vi "Core Logic.vi"(0 "Measurement Context In":refnum<class "Measure Call Context.lvclass">, 5 "Measurement Configuration":T2={"Quick Power Down"=FALSE, "Pin Name"=[], "Source Mode"=[], "Start Value"=[], "Target Value"=[], "Compliance Limit"=[], "Sense Mode"=[], "Default Ramp Rate"=[], "Ramp Rate"=[], "Start Delay"=[], "Relative To"=[], "Transient Response"=[], "Data Capture"=FALSE, "Power line frequency"=1} {"Power line frequency" items=["50 Hz", "60 Hz"]; "Start Value" format="%#_6p"; "Transient Response" items=["Slow", "Normal", "Fast"]; "Sense Mode" items=["Local Sense", "Remote Sense"]; "Relative To" items=["Power sequence start", "Previous source start", "Previous source end"]; "Target Value" format="%#_6p"; "Source Mode" items=["DC Voltage", "DC Current"]; "Start Delay" format="%#_6p"; "Compliance Limit" format="%#_6p"; "Ramp Rate" format="%#_6p"}, 11 "error in":errorcluster) -> (4 "Measurement Context Out":refnum<class "Measure Call Context.lvclass">, 6 "Measurement Results":T1, 15 "error out":errorcluster)   [LabVIEW 2024, in "devicePowerSequencerCoreLogic.lvlib"]
doc: "Use this template to build a producer/consumer design pattern. Use this template when you need to execute a process, such as data analysis, when a data source, such as a triggered acquisition, produces data at an uneven rate and you need to execute the process when the data becomes available."
uses:
  devicePowerSequencerCoreLogic.lvlib
  Measurement Configuration.ctl
  controls/Source Mode.ctl
  controls/Sense Mode.ctl
  controls/Relative To.ctl
  controls/Transient Response.ctl
  controls/Power line frequency.ctl
  Measurement Results.ctl
  <vilib>/Plug-In SDKs/Measurements/Measure Call Context/Measure Call Context.lvclass
  controls/Data Cluster.ctl
  <vilib>/Plug-In SDKs/Clients/Session Management V1/Session Reservation/Session Reservation.lvclass
  controls/Channel Name.ctl
  controls/Software Flags.ctl
  controls/Ramp Configurations.ctl
  controls/Error Info.ctl
  controls/Measurements.ctl
  controls/Voltage and Current Measurements.ctl
  controls/Log Configurations.ctl
  <instrlib>/niDCPower/nidcpower.llb/niDCPower Wait For Event - Event.ctl
  subVIs/Form Error Message.vi/4da3fa3f-d6a2-4c6b-9c9c-fc44bca91f7b.vi
  <vilib>/Plug-In SDKs/Measurements/Measure Call Context/Reserve Sessions - NPin.vi
  <vilib>/Plug-In SDKs/Sessions/niDCPower/Initialize Sessions - NSess.vi
  <vilib>/Plug-In SDKs/Measurements/Measure Call Context/Accessor/Is Canceled.vi
  Device Power Sequencer.lvlib
  <vilib>/Plug-In SDKs/Sessions/niDCPower/NI Session Management niDCPower.lvlib
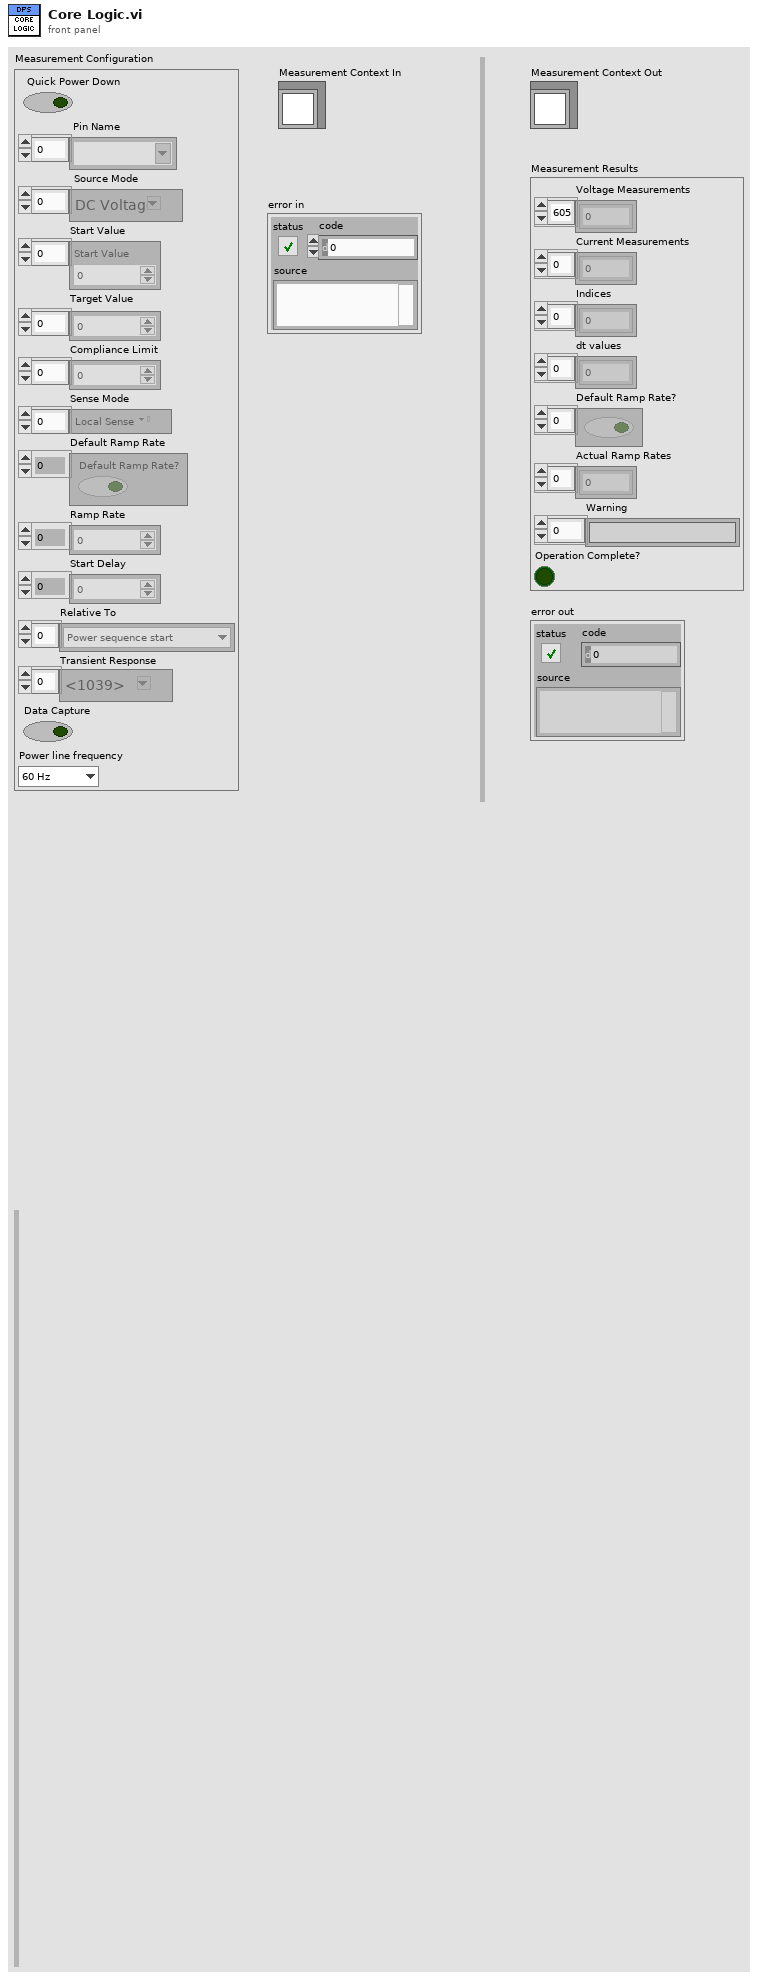
[diagram p1: front panel]
types:
  T1 = typedef "Device Power Sequencer.lvlib/Measurement Results.ctl" = cluster{"Voltage Measurements":dbl[], "Current Measurements":dbl[], "Indices":i32[], "dt values":dbl[], "Default Ramp Rate?":bool[], "Actual Ramp Rates":dbl[], "Warning":string[], "Operation Complete?":bool}
  T2 = typedef "Device Power Sequencer.lvlib/Measurement Configuration.ctl" = cluster{"Quick Power Down":bool, "Pin Name":string[], "Source Mode":T3[], "Start Value":dbl[], "Target Value":dbl[], "Compliance Limit":dbl[], "Sense Mode":T4[], "Default Ramp Rate":bool[], "Ramp Rate":dbl[], "Start Delay":dbl[], "Relative To":T5[], "Transient Response":T6[], "Data Capture":bool, "Power line frequency":T7}
  T3 = typedef "Device Power Sequencer.lvlib/Source Mode.ctl" = i32
  T4 = typedef "Device Power Sequencer.lvlib/Sense Mode.ctl" = i32
  T5 = typedef "Device Power Sequencer.lvlib/Relative To.ctl" = u32
  T6 = typedef "Device Power Sequencer.lvlib/Transient Response.ctl" = i32
  T7 = typedef "Device Power Sequencer.lvlib/Power line frequency.ctl" = u32
  T8 = typedef "devicePowerSequencerCoreLogic.lvlib/Data Cluster.ctl" = cluster{"session reservation":refnum<class "Session Reservation.lvclass">, "measurement context":refnum<class "Measure Call Context.lvclass">, "Measurement Configuration":T2, "Measurement Results":T1, "Channel Settings":T9, "Software Flags":T10, "Ramp Configurations":T11, "Error Info":T12, "Measurements":T13, "Log":T15}
  T9 = typedef "devicePowerSequencerCoreLogic.lvlib/Channel Name.ctl" = cluster{"Channel Name":string[], "Channel Number":string[], "Instrument handle":refnum<k15>[], "Session Exists?":bool[], "Session.name":string[]}
  T10 = typedef "devicePowerSequencerCoreLogic.lvlib/Software Flags.ctl" = cluster{"Initialize Complete?":bool, "Configuration Complete?":bool, "Run Complete?":bool, "Output Complete?":bool, "Safe Power Down In Progress?":bool, "Power Up Operation?":bool, "Canceled?":bool, "Session exists?":bool[], "Advanced Seq Created?":bool[], "Initiated?":bool[], "Unsupported Ramp?":bool[], "Compliance Reached?":bool[], "PowerUp?":bool, "Unsupported Start Delay?":bool[]}
  T11 = typedef "devicePowerSequencerCoreLogic.lvlib/Ramp Configurations.ctl" = cluster{"Minimum Sequence dt(s)":dbl[], "Sequence Delta(s)":dbl[], "Number of steps":i32[], "Actual Ramp Rate(Unit/S)":dbl[], "Total Sequence Time":dbl, "Rising Period":dbl[], "Accumulative Start Delay(s)":dbl[], "Temporary Target Level":dbl[], "Start Level":dbl[], "Measure Period":dbl, "Compliance Skip Duration":dbl[], "Max Sequence Period Index":i32, "Compliance Check Duration":dbl}
  T12 = typedef "devicePowerSequencerCoreLogic.lvlib/Error Info.ctl" = cluster{"Error Occurred?":bool, "Warning List":string[], "Error Phase":string, "Error Code":i32, "error":errorcluster, "Error List":string[], "Custom Error?":bool}
  T13 = typedef "devicePowerSequencerCoreLogic.lvlib/Measurements.ctl" = cluster{"Measurements":T14[], "Calculated Ramp Rate":dbl[], "Default RampRate?":bool[], "Aperture Time":dbl[]}
  T14 = typedef "devicePowerSequencerCoreLogic.lvlib/Voltage and Current Measurements.ctl" = cluster{"Voltage Measurements":dbl[], "Current Measurements":dbl[], "Compliance":bool[]}
  T15 = typedef "devicePowerSequencerCoreLogic.lvlib/Log Configurations.ctl" = cluster{"User Event":refnum<user-event>, "Measure Complete":bool, "Log File Ref.":refnum<file>, "Log Data?":bool, "Async Log Ref.":refnum<vi>}
  T16 = cluster{"Measurment":cluster{"Voltage":dbl[], "Current":dbl[]}[], "Measure Complete?":bool}
  T17 = typedef "niDCPower Wait For Event - Event.ctl" = i32
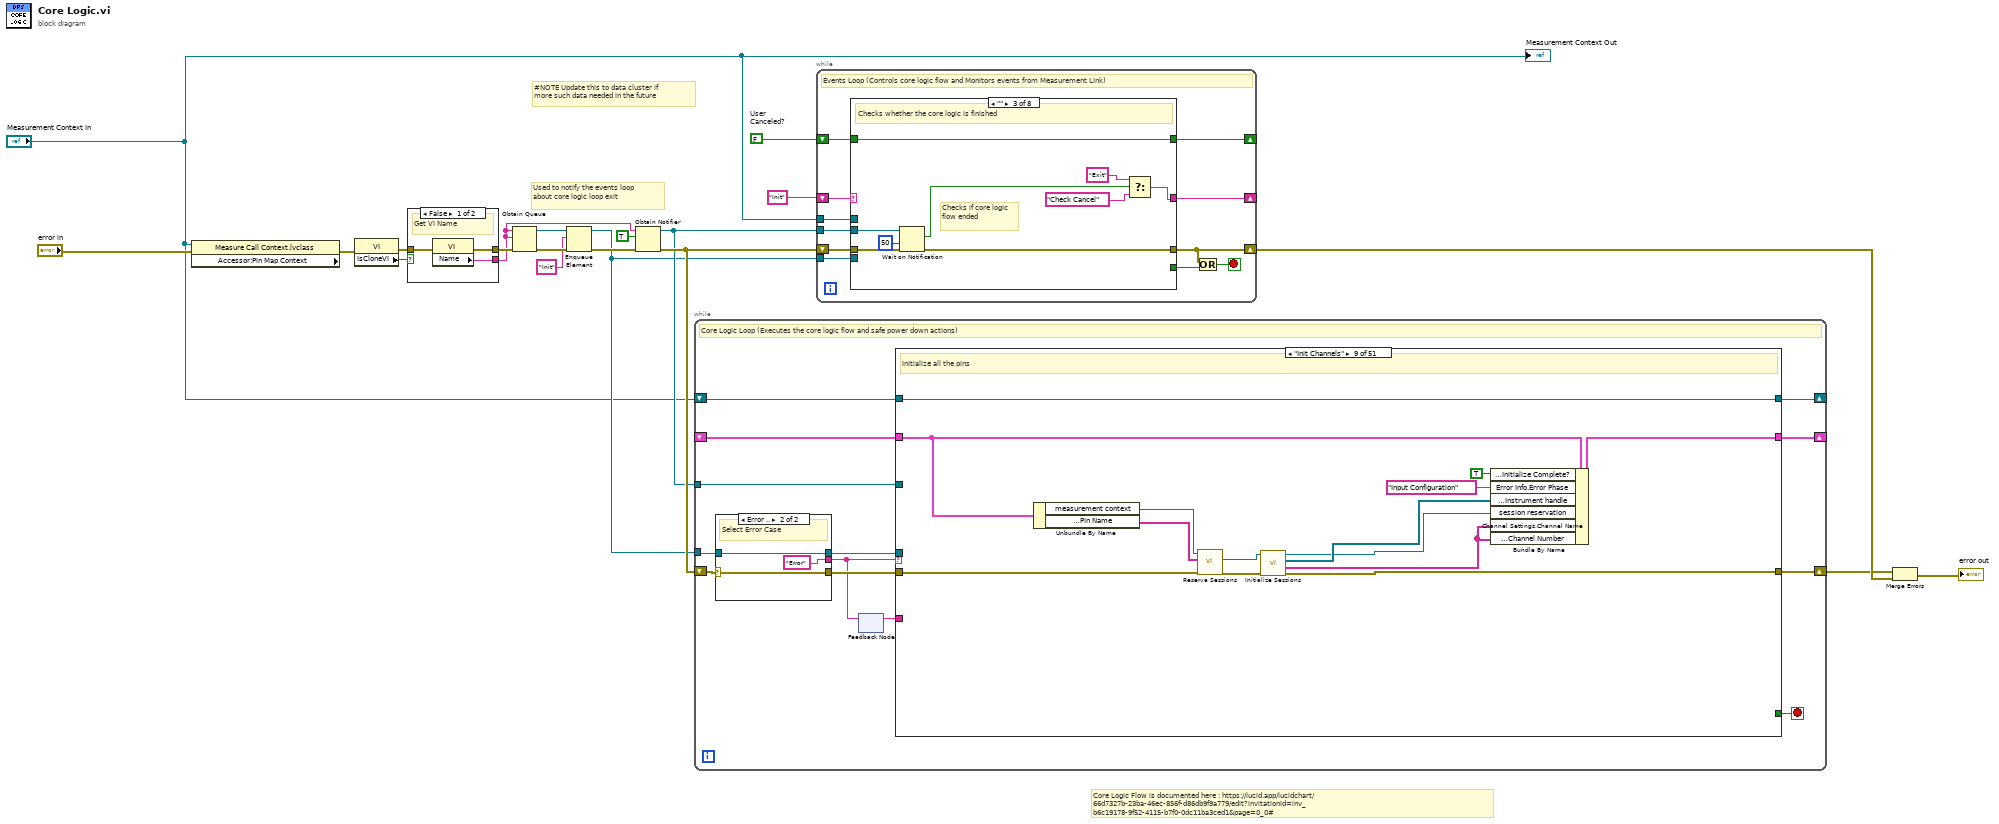
[diagram p0: block diagram]
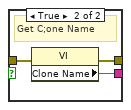
[diagram p2: hidden frame]
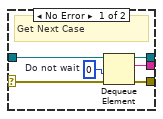
[diagram p3: hidden frame]
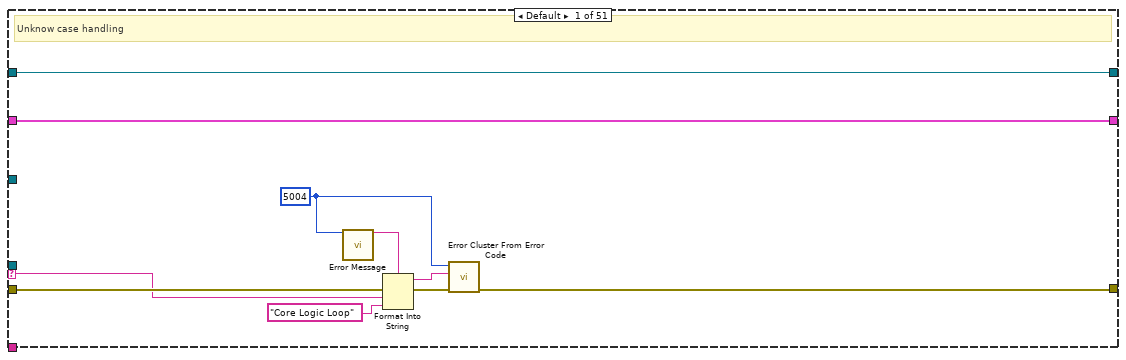
[diagram p4: hidden frame]
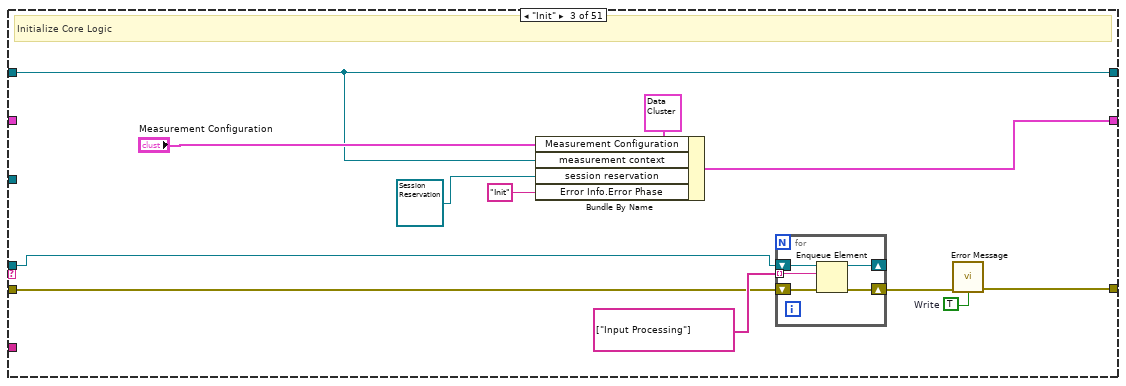
[diagram p6: hidden frame]
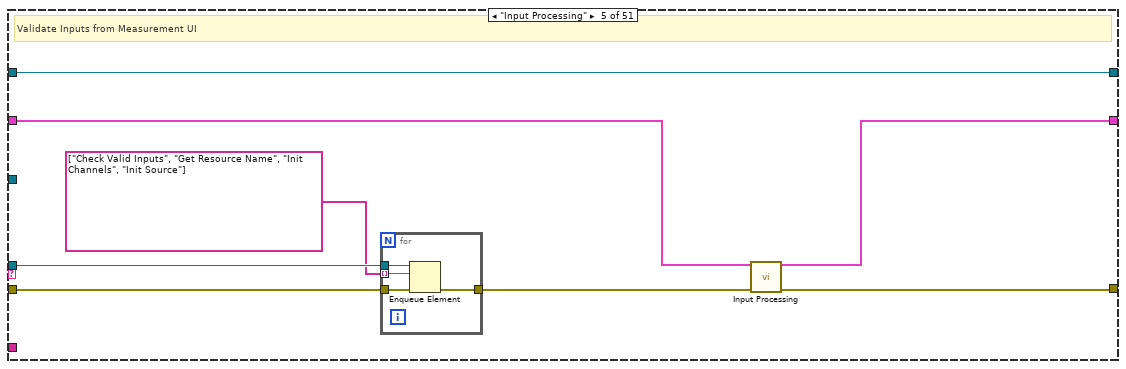
[diagram p8: hidden frame]
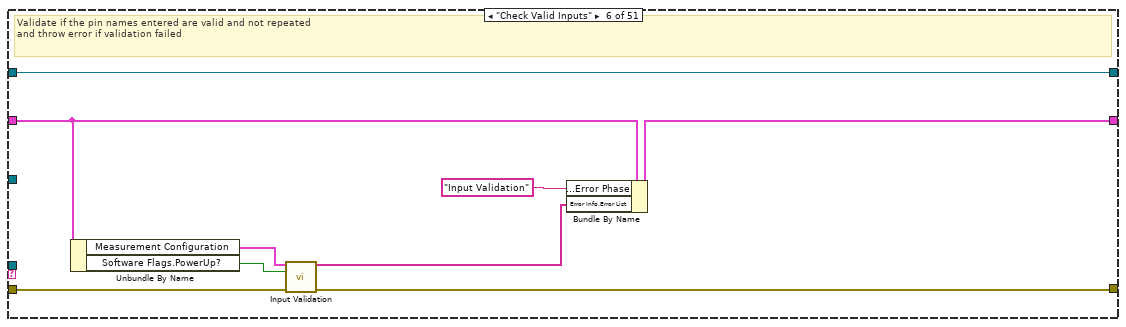
[diagram p9: hidden frame]
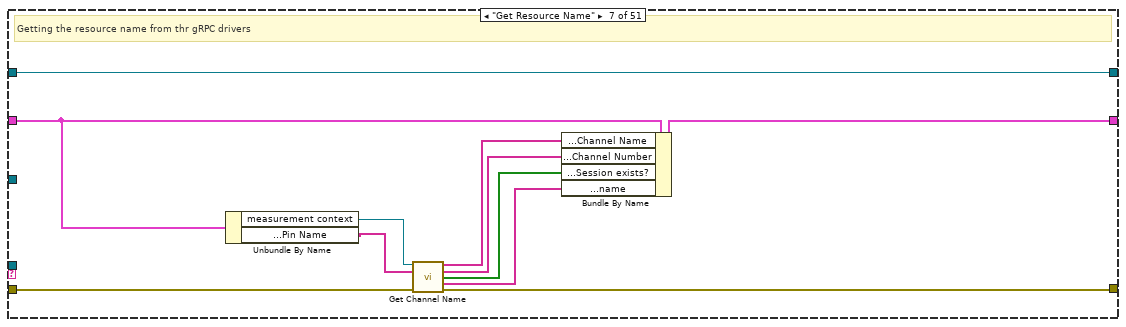
[diagram p10: hidden frame]
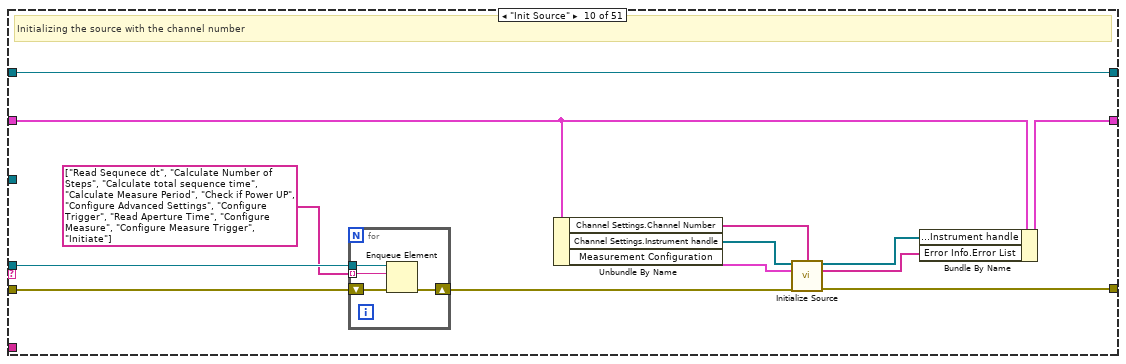
[diagram p12: hidden frame]
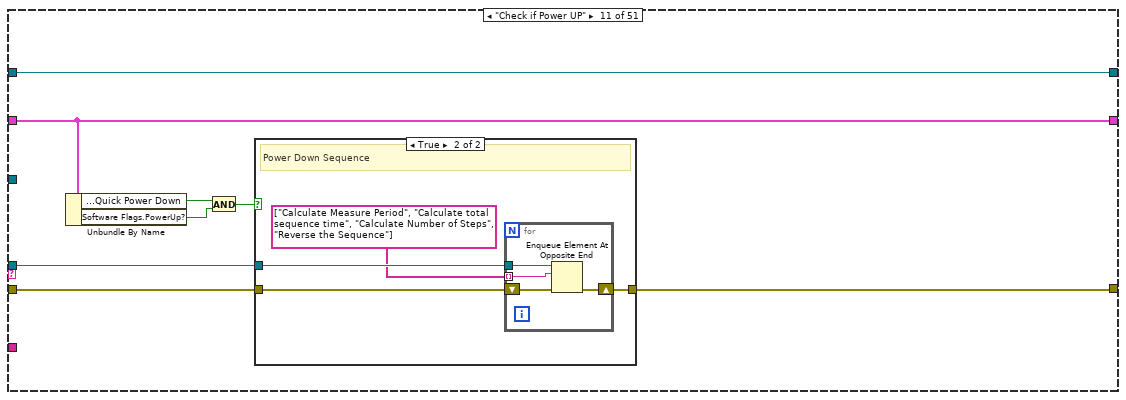
[diagram p13: hidden frame]
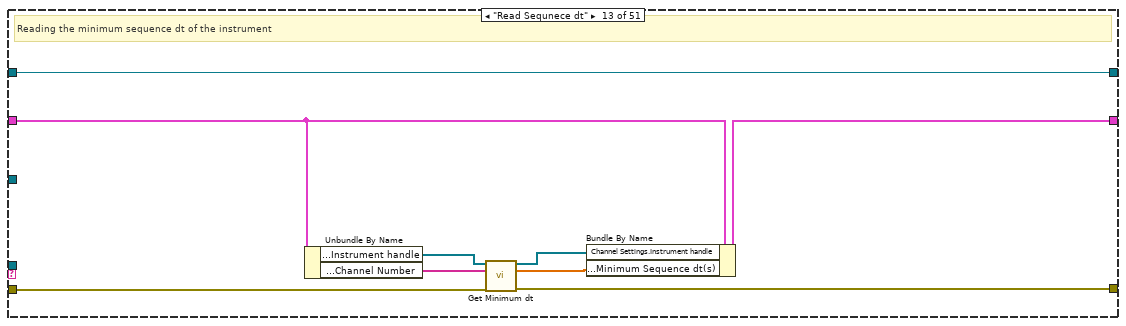
[diagram p16: hidden frame]
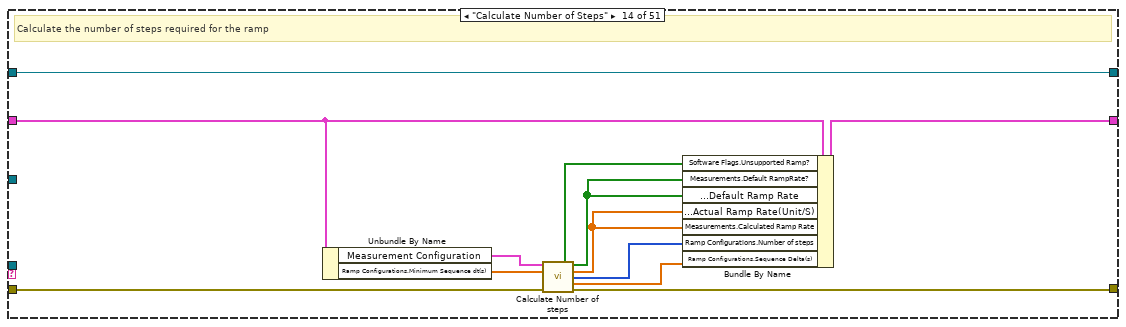
[diagram p17: hidden frame]
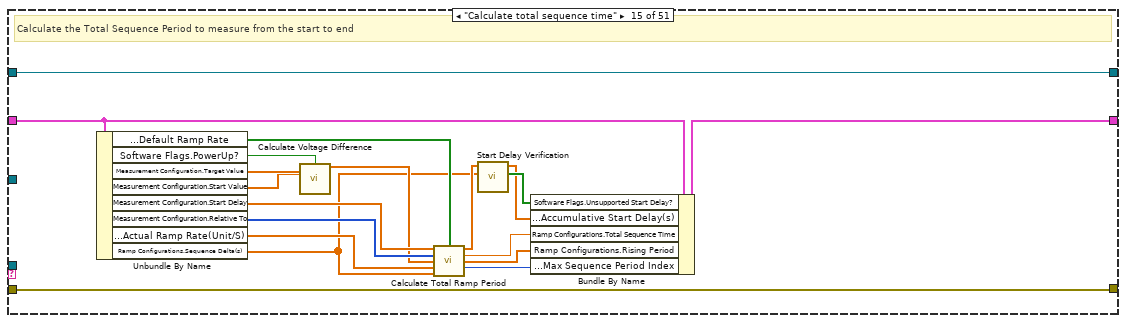
[diagram p18: hidden frame]
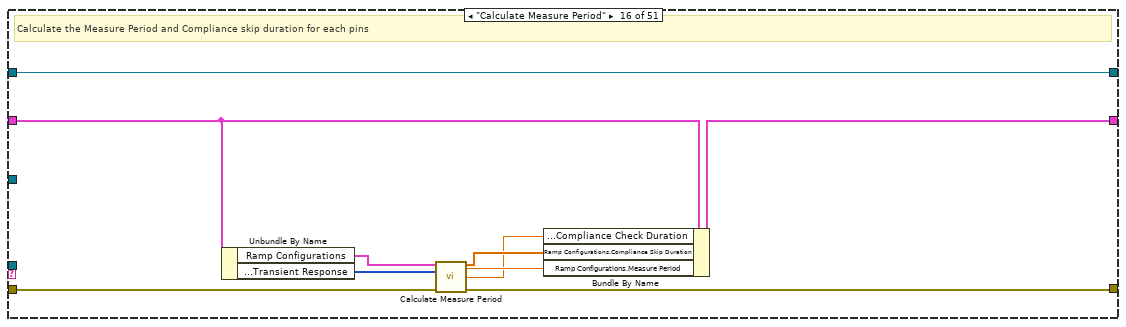
[diagram p19: hidden frame]
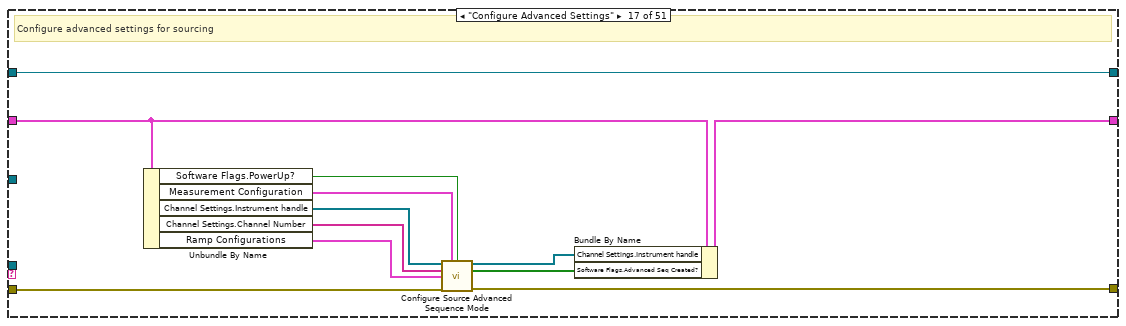
[diagram p20: hidden frame]
diagram:
  w10 = FALSE  # User Canceled?
  # "#NOTE Update this to data cluster if more such data needed in the future"
  # "Core Logic Flow is documented here : https://lucid.app/lucidchart/66d7327b-23ba-46ec-856f-d86db9f9a779/edit?invitationId=inv_b6c19178-9f52-4115-b7f0-0dc11ba3ced1&page=0_0#"
  # "Used to notify the events loop about core logic loop exit"
  n1 = property class="Measure Call Context.lvclass" props=["Accessor:Pin Map Context"](reference="Measurement Context In", error in="error in") -> (error out=w2:errorcluster)  [unwired: 2 out]
  n2 = property class="VI"(error in=w2) -> (error out=w6:errorcluster, "IsCloneVI"=w5:bool)  [unwired: 1 in, 1 out]
  n3 = case shown="False" w5 {
    tunnel: [w23 w25] -> w20
    tunnel: [w22 w24] -> w7
    tunnel: w6 -> [w21 w26]
    frame False {
      # "Get VI Name"
      n4 = property class="VI"(error in=w21) -> (error out=w23:errorcluster, "Name"=w22:string)  [unwired: 1 in, 1 out]
    }
    frame True {
      # "Get C;one Name"
      n5 = property class="VI"(error in=w26) -> (error out=w25:errorcluster, "Clone Name"=w24:string)  [unwired: 1 in, 1 out]
    }
  }
  n6 = Obtain Queue(name (unnamed)=w7, element data type=w7, error in (no error)=w20) -> (queue out=w9:refnum<queue>, error out=w19:errorcluster)  [unwired: 2 in, 1 out]
  n7 = Enqueue Element(queue=w9, element="Init" ("State In"), error in (no error)=w19) -> (queue out=w8:refnum<queue>, error out=w14:errorcluster)  [unwired: 1 in, 1 out]
  n8 = Obtain Notifier(name (unnamed)=w7, notification data type=TRUE, error in (no error)=w14) -> (notifier out=w12:refnum<notifier>, error out=w13:errorcluster)  [unwired: 1 in, 1 out]
  n9 = while {
    shift-right: [w36] -> w4
    shift-left: w13 -> [w38]
    shift-right: [w35] -> _
    shift-left: _ -> [w34]
    tunnel: w12 -> [w33]
    tunnel: w8 -> [w32]
    shift-right: [w27] -> _
    shift-left: "Measurement Context In" -> [w28]
    stop <- w39 stop-if-true
    # "Core Logic Loop (Executes the core logic flow and safe power down actions)"
    n10 = case shown="Error .." w38 {
      selector: w38 -> [w45 w48]
      tunnel: [w44 w48] -> w37
      tunnel: [w43 "Error"] -> w30
      tunnel: w32 -> [w42 w47]
      tunnel: [w40 w47] -> w31
      frame No Error {
        w41 = 0  # Do not wait
        # "Get Next Case"
        n11 = Dequeue Element(queue=w42, timeout in ms (-1)=w41, error in (no error)=w45) -> (queue out=w40:refnum<queue>, element=w43:string, error out=w44:errorcluster)  [unwired: 1 out]
      }
      frame Error {
        # "Select Error Case"
      }
    }
    n12 = feedback-in #1(w30) -> ()
    n13 = feedback #1() -> (w29:string)  [unwired: 1 in]
    n14 = case shown="\"Init Channels\"" w30 {
      selector: w30 -> [w54 _ _ _ _ _ _ _ _ _ _ _ _ _ _ _ _ _ _ _ _ _ _ _ _ _ _ _ _ _ _ _ _ _ _ _ _ _ _ _ _ _ _ _ _ _ _ _ _ _ _]
      tunnel: [_ _ _ _ _ _ _ _ _ _ _ _ _ _ _ _ _ _ _ _ _ _ _ _ _ _ _ _ _ _ _ _ _ _ _ _ _ _ _ _ _ _ _ _ _ _ _ _ _ _ w738] -> w39
      tunnel: w37 -> [w58 w61 w63 w81 w89 w99 w111 w116 w128 w140 w154 w167 w173 w183 w207 w211 w223 w231 w239 w244 w255 w264 w271 w275 w281 w285 w300 w310 w323 w335 w354 w370 w387 w405 w420 w426 w437 w453 w462 w482 w491 w508 w514 w527 w561 w571 w591 w610 w616 w706 w730]
      tunnel: [w56 w61 w67 w81 w84 w100 w112 w116 w129 w137 w152 w167 w174 w182 w207 w210 w224 w232 w239 w243 w256 w265 w271 w274 w280 w284 w297 w310 w318 w335 w360 w370 w383 w411 w420 w422 w438 w453 w461 w483 w486 w509 w514 w520 w561 w572 w592 w610 w622 w705 w717] -> w36
      tunnel: [w57 w60 w71 w80 w85 w98 w110 w115 w127 w142 w155 w166 w172 w186 w203 w214 w222 w236 w238 w245 w258 w268 w270 w273 w279 w287 w291 w309 w327 w334 w342 w367 w382 w413 w419 w425 w436 w452 w464 w480 w493 w511 w513 w532 w560 w570 w595 w609 w617 w704 w719] -> w35
      tunnel: w34 -> [w57 w60 _ w80 w86 w102 w113 w115 w130 w143 w155 w166 w176 w181 w206 w217 w229 w236 w238 w246 w262 w268 w270 w276 w282 w288 w298 w309 w313 w334 w343 w369 w384 w409 w419 w431 w441 w452 w459 w481 w498 w511 w513 w533 w560 w568 w601 w609 w624 w708 w719]
      tunnel: w33 -> [_ _ _ _ _ _ _ _ _ _ _ _ _ _ _ _ _ _ _ _ _ _ _ _ _ _ _ _ _ _ _ _ _ _ _ _ _ _ _ _ _ _ _ _ _ _ _ _ _ _ w736]
      tunnel: w31 -> [_ _ w72 _ w88 _ _ _ _ w141 w153 _ _ _ _ _ _ _ _ _ _ _ _ _ _ w286 _ _ w325 _ w359 _ _ w407 _ _ _ _ w460 _ _ _ _ w529 _ w574 _ _ w621 _ w733]
      tunnel: w29 -> [_ _ _ _ _ _ _ _ _ _ _ _ _ _ _ _ _ _ _ _ _ _ _ _ _ _ _ _ _ _ _ _ _ _ _ _ _ _ _ _ _ _ _ _ _ _ _ _ w612 _ _]
      tunnel: w28 -> [w49 w59 w64 w79 w82 w94 w105 w114 w123 w132 w148 w165 w168 w177 w189 w208 w218 w230 w237 w240 w251 w263 w269 w272 w277 w283 w289 w308 w311 w333 w336 w365 w374 w401 w418 w421 w433 w451 w454 w479 w484 w499 w512 w515 w559 w562 w581 w608 w611 w700 w715]
      tunnel: [w49 w59 w64 w79 w82 w94 w105 w114 w123 w132 w148 w165 w168 w177 w189 w208 w218 w230 w237 w240 w251 w263 w269 w272 w277 w283 w289 w308 w311 w333 w336 w365 w374 w401 w418 w421 w433 w451 w454 w479 w484 w499 w512 w515 w559 w562 w581 w608 w611 w700 w715] -> w27
      frame Default {
        w51 = 5004 ("error code (0)")
        # "Unknow case handling"
        n15 = call "Error Message.vi"("Error Code"=w51) -> ("Error Message"=w50:string)  [unwired: 12 in, 2 out]
        n16 = Format Into String(format string=w50, error in=w58, w54, "Core Logic Loop" ("input 2")) -> (resulting string=w53:string, error out=w55:errorcluster)  [unwired: 1 in]
        n17 = call <vilib>:"Error Cluster From Error Code.vi"("error in (no error)"=w55, "error message (\"\")"=w53, "error code (0)"=w51) -> ("error out"=w56:errorcluster)  [unwired: 6 in]
      }
      frame "----------------- INITIALIZE -----------------" {
      }
      frame "Init" {
        w70 = TRUE  # Write
        # "Initialize Core Logic"
        n18 = Bundle By Name(cluster=T8 {"session reservation"=refnum, "measurement context"=refnum, "Measurement Configuration"={"Quick Power Down"=FALSE, "Pin Name"=[], "Source Mode"=[], "Start Value"=[], "Target Value"=[], "Compliance Limit"=[], "Sense Mode"=[], "Default Ramp Rate"=[], "Ramp Rate"=[], "Start Delay"=[], "Relative To"=[], "Transient Response"=[], "Data Capture"=FALSE, "Power line frequency"=1}, "Measurement Results"={"Voltage Measurements"=[], "Current Measurements"=[], "Indices"=[], "dt values"=[], "Default Ramp Rate?"=[], "Actual Ramp Rates"=[], "Warning"=[], "Operation Complete?"=FALSE}, "Channel Settings"={"Channel Name"=[], "Channel Number"=[], "Instrument handle"=[], "Session Exists?"=[], "Session.name"=[]}, "Software Flags"={"Initialize Complete?"=FALSE, "Configuration Complete?"=FALSE, "Run Complete?"=FALSE, "Output Complete?"=FALSE, "Safe Power Down In Progress?"=FALSE, "Power Up Operation?"=FALSE, "Canceled?"=FALSE, "Session exists?"=[], "Advanced Seq Created?"=[], "Initiated?"=[], "Unsupported Ramp?"=[], "Compliance Reached?"=[], "PowerUp?"=FALSE, "Unsupported Start Delay?"=[]}, "Ramp Configurations"={"Minimum Sequence dt(s)"=[], "Sequence Delta(s)"=[], "Number of steps"=[], "Actual Ramp Rate(Unit/S)"=[], "Total Sequence Time"=0.0, "Rising Period"=[], "Accumulative Start Delay(s)"=[], "Temporary Target Level"=[], "Start Level"=[], "Measure Period"=0.0, "Compliance Skip Duration"=[], "Max Sequence Period Index"=0, "Compliance Check Duration"=0.0}, "Error Info"={"Error Occurred?"=FALSE, "Warning List"=[], "Error Phase"="", "Error Code"=5100, "error"={"status"=FALSE, "code"=0, "source"=""}, "Error List"=[], "Custom Error?"=FALSE}, "Measurements"={"Measurements"=[], "Calculated Ramp Rate"=[], "Default RampRate?"=[], "Aperture Time"=[]}, "Log"={"User Event"=refnum, "Measure Complete"=FALSE, "Log File Ref."=refnum, "Log Data?"=FALSE, "Async Log Ref."=refnum}} ("Data Cluster"), "Measurement Configuration"="Measurement Configuration", "measurement context"=w64, "session reservation"=refnum<class "Session Reservation.lvclass"> refnum, "Error Info.Error Phase"="Init") -> (w71:T8)
        n19 = for {
          shift-right: [w76] -> w69
          shift-left: w63 -> [w78]
          shift-right: [w75] -> _
          shift-left: w72 -> [w77]
          tunnel: string[] ["Input Processing"] -> [w74] mode=indexing
          n20 = Enqueue Element(queue=w77, element=w74, error in (no error)=w78) -> (queue out=w75:refnum<queue>, error out=w76:errorcluster)  [unwired: 1 in, 1 out]
        }
        n21 = call "Error Message.vi"("error in (no error)"=w69, "ReadError?F:T"=w70) -> ("error out"=w67:errorcluster)  [unwired: 11 in, 2 out]
      }
      frame "---------------------VALIDATION---------------------" {
      }
      frame "Input Processing" {
        # "Validate Inputs from Measurement UI"
        n22 = for {
          tunnel: string[] ["Check Valid Inputs", "Get Resource Name", "Init Channels", "Init Source"] ("State In") -> [w92] mode=indexing
          tunnel: w88 -> [w90]
          tunnel: w89 -> [w91]
          tunnel: [w93] -> w83
          n23 = Enqueue Element(queue=w90, element=w92, error in (no error)=w91) -> (error out=w93:errorcluster)  [unwired: 1 in, 2 out]
        }
        n24 = call "Input Processing.vi"("Data Cluster"=w86, "error in (no error)"=w83) -> ("Data Cluster OUT"=w85:T8, "error out"=w84:errorcluster)  [unwired: 12 in]
      }
      frame "Check Valid Inputs" {
        # "Validate if the pin names entered are valid and not repeated\nand throw error if validation failed"
        n25 = Unbundle By Name(w102) -> ("Measurement Configuration"=w101:T2, "Software Flags.PowerUp?"=w95:bool)
        n26 = call "Input Validation.vi"("Measurement Configuration"=w101, "PowerUP?"=w95, "error in (no error)"=w99) -> ("Error"=w96:string[], "error out"=w100:errorcluster)  [unwired: 11 in]
        n27 = Bundle By Name(cluster=w102, "Error Info.Error Phase"="Input Validation", "Error Info.Error List"=w96) -> (w98:T8)
      }
      frame "Get Resource Name" {
        # "Getting the resource name from thr gRPC drivers"
        n28 = Unbundle By Name(w113) -> ("measurement context"=w104:refnum<class "Measure Call Context.lvclass">, "Measurement Configuration.Pin Name"=w103:string[])
        n29 = call "Get Channel Name.vi"("measurement context in"=w104, "Pin Name[]"=w103, "error in (no error)"=w111) -> ("Channel Name"=w109:string[], "Channel Number"=w108:string[], "Session Exists"=w107:bool[], "Session.name"=w106:string[], "error out"=w112:errorcluster)  [unwired: 8 in]
        n30 = Bundle By Name(cluster=w113, "Channel Settings.Channel Name"=w109, "Channel Settings.Channel Number"=w108, "Software Flags.Session exists?"=w107, "Channel Settings.Session.name"=w106) -> (w110:T8)
      }
      frame "----------------SESSION INIT------------------" {
      }
      frame "Init Channels" {
        # "Initialize all the pins"
        n31 = Unbundle By Name(w130) -> ("measurement context"=w122:refnum<class "Measure Call Context.lvclass">, "Measurement Configuration.Pin Name"=w124:string[])
        n32 = call-poly <vilib>:"Reserve Sessions.vi"("error in"=w128, "pin or relay names"=w124, "measurement context in"=w122) -> ("error out"=w117:errorcluster, "session reservation out"=w118:refnum<class "Session Reservation.lvclass">)  [unwired: 6 in, 1 out]
        n33 = call-poly <vilib>:"Initialize Sessions.vi"("error in"=w117, "session reservation in"=w118) -> ("error out"=w129:errorcluster, "channel lists"=w119:string[], "sessions"=w121:refnum<k15>[], "session reservation out"=w120:refnum<class "Session Reservation.lvclass">)  [unwired: 6 in]
        n34 = Bundle By Name(cluster=w130, "Software Flags.Initialize Complete?"=TRUE, "Error Info.Error Phase"="Input Configuration", "Channel Settings.Instrument handle"=w121, "session reservation"=w120, "Channel Settings.Channel Name"=w119, "Channel Settings.Channel Number"=w119) -> (w127:T8)
      }
      frame "Init Source" {
        # "Initializing the source with the channel number"
        n35 = for {
          tunnel: w141 -> [w147]
          shift-right: [w145] -> w139
          shift-left: w140 -> [w146]
          tunnel: string[] ["Read Sequnece dt", "Calculate Number of Steps", "Calculate total sequence time", "Calculate Measure Period", "Check if Power UP", "Configure Advanced Settings", "Configure Trigger", "Read Aperture Time", "Configure Measure", "Configure Measure Trigger", "Initiate"] -> [w144] mode=indexing
          n36 = Enqueue Element(queue=w147, element=w144, error in (no error)=w146) -> (error out=w145:errorcluster)  [unwired: 1 in, 2 out]
        }
        n37 = Unbundle By Name(w143) -> ("Channel Settings.Channel Number"=w131:string[], "Channel Settings.Instrument handle"=w136:refnum<k15>[], "Measurement Configuration"=w135:T2)
        n38 = call "Initialize Source.vi"("Intrument Handle[]"=w136, "Channel Number"=w131, "Measurement Configuration"=w135, "error in (no error)"=w139) -> ("Intrument Handle out[]"=w134:refnum<k15>[], "Error"=w133:string[], "error out"=w137:errorcluster)  [unwired: 9 in]
        n39 = Bundle By Name(cluster=w143, "Channel Settings.Instrument handle"=w134, "Error Info.Error List"=w133) -> (w142:T8)
      }
      frame "Check if Power UP" {
        n40 = Unbundle By Name(w155) -> ("Measurement Configuration.Quick Power Down"=w150:bool, "Software Flags.PowerUp?"=w149:bool)
        n41 = And(x=w150, y=w149) -> (x .and. y?=w151:bool)
        n42 = case shown="True" w151 {
          tunnel: w154 -> [w156 w160]
          tunnel: w153 -> [_ w159]
          tunnel: [w156 w158] -> w152
          frame False {
            # "Power UP Sequence"
          }
          frame True {
            # "Power Down Sequence"
            n43 = for {
              tunnel: w159 -> [w163]
              shift-right: [w162] -> w158
              shift-left: w160 -> [w164]
              tunnel: string[] ["Calculate Measure Period", "Calculate total sequence time", "Calculate Number of Steps", "Reverse the Sequence"] -> [w161] mode=indexing
              n44 = Enqueue Element At Opposite End(queue=w163, element=w161, error in (no error)=w164) -> (error out=w162:errorcluster)  [unwired: 1 in, 2 out]
            }
          }
        }
      }
      frame "-------------- SOURCE CONFIGURATIONS --------------" {
      }
      frame "Read Sequnece dt" {
        # "Reading the minimum sequence dt of the instrument"
        n45 = Unbundle By Name(w176) -> ("Channel Settings.Instrument handle"=w175:refnum<k15>[], "Channel Settings.Channel Number"=w169:string[])
        n46 = call "Get Minimum dt.vi"("Instrument handle IN"=w175, "Channel Number"=w169, "error in (no error)"=w173) -> ("Instrument handle OUT"=w171:refnum<k15>[], "Minimum dt"=w170:dbl[], "error out"=w174:errorcluster)  [unwired: 10 in]
        n47 = Bundle By Name(cluster=w176, "Channel Settings.Instrument handle"=w171, "Ramp Configurations.Minimum Sequence dt(s)"=w170) -> (w172:T8)
      }
      frame "Calculate Number of Steps" {
        # "Calculate the number of steps required for the ramp"
        n48 = Unbundle By Name(w181) -> ("Measurement Configuration"=w188:T2, "Ramp Configurations.Minimum Sequence dt(s)"=w187:dbl[])
        n49 = call "Calculate Number of steps.vi"("Measurement Configuration"=w188, "Minimum Sequence Delta"=w187, "error in (no error)"=w183) -> ("Unsupported Ramp?"=w180:bool[], "Default Ramp Rate?"=w179:bool[], "Actual Ramp Rate[]"=w178:dbl[], "Number of steps[]"=w185:i32[], "Sequnence Delta[]"=w184:dbl[], "error out"=w182:errorcluster)  [unwired: 7 in]
        n50 = Bundle By Name(cluster=w181, "Software Flags.Unsupported Ramp?"=w180, "Measurements.Default RampRate?"=w179, "Measurement Configuration.Default Ramp Rate"=w179, "Ramp Configurations.Actual Ramp Rate(Unit/S)"=w178, "Measurements.Calculated Ramp Rate"=w178, "Ramp Configurations.Number of steps"=w185, "Ramp Configurations.Sequence Delta(s)"=w184) -> (w186:T8)
      }
      frame "Calculate total sequence time" {
        # "Calculate the Total Sequence Period to measure from the start to end"
        n51 = Unbundle By Name(w206) -> ("Measurement Configuration.Default Ramp Rate"=w194:bool[], "Software Flags.PowerUp?"=w198:bool, "Measurement Configuration.Target Value"=w197:dbl[], "Measurement Configuration.Start Value"=w196:dbl[], "Measurement Configuration.Start Delay"=w205:dbl[], "Measurement Configuration.Relative To"=w201:T5[], "Ramp Configurations.Actual Ramp Rate(Unit/S)"=w204:dbl[], "Ramp Configurations.Sequence Delta(s)"=w190:dbl[])
        n52 = call "Calculate Voltage Difference.vi"("Target Value"=w197, "PowerUp?"=w198, "Start Value"=w196) -> ("Value  difference"=w199:dbl[])  [unwired: 12 in]
        n53 = call "Calculate Total Ramp Period.vi"("Start Delay In"=w205, "Default Ramp Rate"=w194, "Relative To"=w201, "Level"=w199, "Ramp Rate"=w204, "Sequence Delta"=w190) -> ("Accumulative Start delays"=w192:dbl[], "Total Power Seq Period"=w200:dbl, "Rising Period"=w202:dbl[], "Max Sequence Period Index"=w195:i32)  [unwired: 6 in]
        n54 = call "Start Delay Verification.vi"("Minimum sequence step dt"=w190, "Start delays"=w192) -> ("Unsupported Start Delay?"=w193:bool[], "Start delays"=w191:dbl[])  [unwired: 8 in]
        n55 = Bundle By Name(cluster=w206, "Software Flags.Unsupported Start Delay?"=w193, "Ramp Configurations.Accumulative Start Delay(s)"=w191, "Ramp Configurations.Total Sequence Time"=w200, "Ramp Configurations.Rising Period"=w202, "Ramp Configurations.Max Sequence Period Index"=w195) -> (w203:T8)
      }
      frame "Calculate Measure Period" {
        # "Calculate the Measure Period and Compliance skip duration for each pins"
        n56 = Unbundle By Name(w217) -> ("Ramp Configurations"=w216:T11, "Measurement Configuration.Transient Response"=w215:T6[])
        n57 = call "Calculate Measure Period.vi"("Ramp Configurations"=w216, "Transient Response"=w215, "error in (no error)"=w211) -> ("Compliance Skip Duration"=w213:dbl[], "Measure Period"=w212:dbl, "Compliance Check Duration"=w209:dbl, "error out"=w210:errorcluster)  [unwired: 9 in]
        n58 = Bundle By Name(cluster=w217, "Ramp Configurations.Compliance Check Duration"=w209, "Ramp Configurations.Compliance Skip Duration"=w213, "Ramp Configurations.Measure Period"=w212) -> (w214:T8)
      }
      frame "Configure Advanced Settings" {
        # "Configure advanced settings for sourcing"
        n59 = Unbundle By Name(w229) -> ("Software Flags.PowerUp?"=w219:bool, "Measurement Configuration"=w228:T2, "Channel Settings.Instrument handle"=w227:refnum<k15>[], "Channel Settings.Channel Number"=w226:string[], "Ramp Configurations"=w225:T11)
        n60 = call "Configure Source Advanced Sequence Mode.vi"("Instrument handle IN"=w227, "Measurement Configuration"=w228, "PowerUP?"=w219, "Channel Number"=w226, "Ramp Configurations"=w225, "error in (no error)"=w223) -> ("Instrument Handle OUT"=w221:refnum<k15>[], "Advance Seq Created?"=w220:bool[], "error out"=w224:errorcluster)  [unwired: 7 in]
        n61 = Bundle By Name(cluster=w229, "Channel Settings.Instrument handle"=w221, "Software Flags.Advanced Seq Created?"=w220) -> (w222:T8)
      }
      frame "Configure Trigger" {
        # "Configure the start trigger for all pins"
        n62 = Unbundle By Name(w236) -> ("Channel Settings.Instrument handle"=w235:refnum<k15>[], "Channel Settings.Channel Number"=w234:string[], "Measurement Configuration.Relative To"=w233:T5[])
        n63 = call "Configure Trigger.vi"("Instrument handles in"=w235, "Channels Name"=w234, "Relative To"=w233, "error in (no error)"=w231) -> ("error out"=w232:errorcluster)  [unwired: 11 in]
      }
      frame "--------------MEASURE CONFIGURATIONS---------------" {
      }
      frame "Read Aperture Time" {
        # "Reading the minimum Aperture Time of the instrument"
        n64 = Unbundle By Name(w246) -> ("Channel Settings.Instrument handle"=w250:refnum<k15>[], "Channel Settings.Channel Number"=w247:string[], "Ramp Configurations.Minimum Sequence dt(s)"=w242:dbl[], "Ramp Configurations.Measure Period"=w241:dbl)
        n65 = call "Get Aperture Time.vi"("Instrument handle IN"=w250, "Channel Name"=w247, "Minimum Sequence dt(s)"=w242, "Measure Period"=w241, "error in (no error)"=w244) -> ("Instrument handle OUT"=w249:refnum<k15>[], "Aperture Time"=w248:dbl[], "error out"=w243:errorcluster)  [unwired: 8 in]
        n66 = Bundle By Name(cluster=w246, "Channel Settings.Instrument handle"=w249, "Measurements.Aperture Time"=w248) -> (w245:T8)
      }
      frame "Configure Measure" {
        # "Configure the settings to measure Voltage and current"
        n67 = Unbundle By Name(w262) -> ("Measurements.Aperture Time"=w252:dbl[], "Channel Settings.Instrument handle"=w261:refnum<k15>[], "Channel Settings.Channel Number"=w260:string[], "Ramp Configurations.Measure Period"=w259:dbl, "Measurement Configuration"=w253:T2)
        n68 = call "Measure configuration.vi"("Intrument Handle[]"=w261, "Aperture Time"=w252, "Channel Name"=w260, "Measure Period"=w259, "Measurement Configuration"=w253, "error in (no error)"=w255) -> ("Intrument Handle out[]"=w257:refnum<k15>[], "Aperture Time"=w254:dbl[], "error out"=w256:errorcluster)  [unwired: 7 in]
        n69 = Bundle By Name(cluster=w262, "Channel Settings.Instrument handle"=w257, "Measurements.Aperture Time"=w254) -> (w258:T8)
      }
      frame "Configure Measure Trigger" {
        # "Configure the measure trigger to measure the voltage"
        n70 = Unbundle By Name(w268) -> ("Channel Settings.Instrument handle"=w267:refnum<k15>[], "Channel Settings.Channel Number"=w266:string[])
        n71 = call "Measure Trigger.vi"("Intrument Handle[]"=w267, "Channel Name"=w266, "error in (no error)"=w264) -> ("error out"=w265:errorcluster)  [unwired: 12 in]
      }
      frame "---------------DATA LOGGER---------------" {
      }
      frame "Init Logger" {
        # "Create Data Logger"
        n72 = call "Initialize Logger.vi"("error in (no error)"=w275, "Data Cluster OUT in"=w276) -> ("error out"=w274:errorcluster, "Data Cluster OUT out"=w273:T8)  [unwired: 8 in]
      }
      frame "Log Measure Configuration" {
        # "Log Measurment Configurations & Results"
        n73 = control-ref of="Measurement Configuration"() -> (w278:refnum<vi>)
        n74 = call "Log Measurment Configurations.vi"("Data Cluster OUT in"=w282, "Cluster in"=w278, "error in (no error)"=w281) -> ("Data Cluster OUT out"=w279:T8, "error out"=w280:errorcluster)  [unwired: 6 in]
      }
      frame "Start Async Log" {
        # "Run the Asyncronus Logger VI"
        n75 = call "Start Asynchronus Logger.vi"("error in (no error)"=w285, "Queue in"=w286, "Data Cluster OUT in"=w288) -> ("error out"=w284:errorcluster, "Data Cluster OUT out"=w287:T8)  [unwired: 7 in]
      }
      frame "Stop Logger" {
        # "#dlogchange"
        # "Stop execution of Async Logger"
        n76 = Unbundle By Name(w298) -> ("Log.Log Data?"=w294:bool, "Log.User Event"=w296:refnum<user-event>)
        n77 = Not A Number/Path/Refnum?(number/path/refnum=w296) -> (NaN/Path/Refnum?=w295:bool)
        n78 = Not(x=w295) -> (.not. x?=w292:bool)
        n79 = And(x=w294, y=w292) -> (x .and. y?=w293:bool)
        n80 = case shown="True" w293 {
          tunnel: w296 -> [_ w307]
          tunnel: w300 -> [w301 w303]
          tunnel: [w301 w302] -> w299
          frame False {
          }
          frame True {
            w306 = T16 {"Measurment"=[], "Measure Complete?"=FALSE}  # Log Event Data
            n81 = Bundle By Name(cluster=w306, "Measure Complete?"=TRUE) -> (w304:T16)
            n82 = Generate User Event(user event=w307, event data cluster=w304, error in=w303) -> (error out=w302:errorcluster)  [unwired: 1 in, 1 out]
          }
        }
        n83 = Bundle By Name(cluster=w298, "Log.Log Data?"=FALSE) -> (w291:T8)
        n84 = call <vilib>:"Clear Errors.vi"("error in (no error)"=w299) -> ("error out"=w297:errorcluster)  [unwired: 5 in, 1 out]
      }
      frame "---------------- START POWERUP/DOWN ------------------" {
      }
      frame "Initiate" {
        # "Initiate all the pins to start sourcing"
        n85 = Unbundle By Name(w313) -> ("Measurement Configuration.Data Capture"=w314:bool)
        n86 = Select(t=string[] ["Init Logger", "Log Measure Configuration", "Start Async Log", "Measure"], s=w314, f=string[] ["Measure"]) -> (s? t:f=w315:string[])
        n87 = for {
          tunnel: w325 -> [w332]
          shift-right: [w330] -> w324
          shift-left: w323 -> [w331]
          tunnel: w315 -> [w329] mode=indexing
          n88 = Enqueue Element(queue=w332, element=w329, error in (no error)=w331) -> (error out=w330:errorcluster)  [unwired: 1 in, 2 out]
        }
        n89 = Unbundle By Name(w313) -> ("Error Info.Error Occurred?"=w319:bool, "Error Info.Error Phase"=w321:string, "Channel Settings.Instrument handle"=w328:refnum<k15>[], "Channel Settings.Channel Number"=w312:string[])
        n90 = call "Initiate Powerup.vi"("Instrument handles in"=w328, "Channel Name"=w312, "error in (no error)"=w324) -> ("Initiated?"=w326:bool[], "error out"=w318:errorcluster)  [unwired: 11 in]
        n91 = Select(t=w321, s=w319, f="Power UP" ("Error Info.Error Phase")) -> (s? t:f=w320:string)
        n92 = Bundle By Name(cluster=w313, "Error Info.Error Phase"=w320, "Software Flags.Initiated?"=w326) -> (w327:T8)
      }
      frame "-------------------- OUTPUT---------------------" {
      }
      frame "Measure" {
        # "Fetch the data from theSMU Buffer"
        n93 = Unbundle By Name(w343) -> ("Ramp Configurations.Compliance Check Duration"=w337:dbl, "Error Info.Error List"=w341:string[], "Measurements.Measurements"=w350:T14[], "Channel Settings.Instrument handle"=w352:refnum<k15>[], "Channel Settings.Channel Number"=w351:string[], "Ramp Configurations.Compliance Skip Duration"=w349:dbl[], "Measurements.Aperture Time"=w348:dbl[], "Measurement Configuration.Pin Name"=w347:string[], "Log"=w338:T15)
        n94 = call "Measure.vi"("Instrument handle"=w352, "Measurements"=w350, "Compliance Check Duration"=w337, "Channel Name"=w351, "Compliance Skip Duration"=w349, "Aperture Time"=w348, "error in (no error)"=w354, "Pin Name"=w347, "Log Configurations"=w338) -> ("Measurements"=w344:T14[], "Measure complete?"=w346:bool[], "Error List[]"=w340:string[], "error out"=w353:errorcluster)  [unwired: 3 in]
        n95 = Insert Into Array(array=w341, new element=w340) -> (w339:string[])  [unwired: 1 in]
        n96 = And Array Elements(Boolean array=w346) -> (logical AND=w355:bool)
        n97 = Bundle By Name(cluster=w343, "Error Info.Error Phase"="Measure", "Error Info.Error List"=w339, "Measurements.Measurements"=w344) -> (w342:T8)
        n98 = Select(t=string[] ["Verify Sequence", "Check Compliance", "Output Processing"], s=w355, f=string[] ["Measure"]) -> (s? t:f=w357:string[])
        n99 = for {
          tunnel: w359 -> [w364]
          shift-right: [w362] -> w360
          shift-left: w353 -> [w363]
          tunnel: w357 -> [w361] mode=indexing
          n100 = Enqueue Element(queue=w364, element=w361, error in (no error)=w363) -> (error out=w362:errorcluster)  [unwired: 1 in, 2 out]
        }
      }
      frame "Check Compliance" {
        # "Checks compliance reached momentarily"
        n101 = Unbundle By Name(w369) -> ("Measurements.Measurements"=w368:T14[])
        n102 = for {
          tunnel: w368 -> [w373] mode=indexing
          tunnel: [w371] -> w366 mode=indexing
          n103 = Unbundle By Name(w373) -> ("Compliance"=w372:bool[])
          n104 = Or Array Elements(Boolean array=w372) -> (logical OR=w371:bool)
        }
        n105 = Bundle By Name(cluster=w369, "Software Flags.Compliance Reached?"=w366) -> (w367:T8)
      }
      frame "Verify Sequence" {
        # "Checks Powerup successfull or not"
        n106 = Unbundle By Name(w384) -> ("Error Info.Error List"=w378:string[], "Measurement Configuration.Quick Power Down"=w376:bool, "Software Flags.PowerUp?"=w375:bool, "Measurement Configuration"=w386:T2, "Measurements"=w385:T13)
        n107 = case "Power Down?" shown="True" w375 {
          tunnel: [TRUE ("Power Down") w389] -> w377
          tunnel: w376 -> [_ w389]
          frame False {
            # "Power Down"
          }
          frame True {
            # "Power Up"
          }
        }
        n108 = case shown="True" w377 {
          tunnel: w387 -> [w394 w400]
          tunnel: w386 -> [w393 w397]
          tunnel: w385 -> [w392 w398]
          tunnel: [w391 w399] -> w383
          tunnel: [w390 w396] -> w379
          tunnel: w375 -> [_ w395]
          frame False {
            # "Powerup"
            n109 = call "Verify powerup.vi"("Measurement Configuration"=w393, "Measurements"=w392, "error in (no error)"=w394) -> ("Error[]"=w390:string[], "error out"=w391:errorcluster)  [unwired: 11 in]
          }
          frame True {
            # "Powerdown"
            n110 = call "Verify Power Down.vi"("Measurement Configuration"=w397, "Measurements"=w398, "PowerUP?"=w395, "error in (no error)"=w400) -> ("Error[]"=w396:string[], "error out"=w399:errorcluster)  [unwired: 10 in]
          }
        }
        n111 = Insert Into Array(array=w378, new element=w379) -> (w380:string[])  [unwired: 1 in]
        n112 = Bundle By Name(cluster=w384, "Error Info.Error Phase"="Verify Sequence", "Error Info.Error List"=w380) -> (w382:T8)
      }
      frame "Output Processing" {
        # "Process the outputs to be sent to the UI/Teststand"
        n113 = for {
          tunnel: w407 -> [w417]
          shift-right: [w415] -> w406
          shift-left: w405 -> [w416]
          tunnel: string[] ["Abort session", "Close Instrument Handle", "Exit"] -> [w414] mode=indexing
          n114 = Enqueue Element(queue=w417, element=w414, error in (no error)=w416) -> (error out=w415:errorcluster)  [unwired: 1 in, 2 out]
        }
        n115 = Unbundle By Name(w409) -> ("Measurements"=w408:T13, "Software Flags"=w403:T10, "Measurement Configuration.Quick Power Down"=w402:bool)
        n116 = call "Output Processing.vi"("Measurements"=w408, "Software Flags"=w403, "Powerdown?"=w402, "error in (no error)"=w406) -> ("Measurement Results"=→"Measurement Results":T1, "error out"=w411:errorcluster)  [unwired: 10 in]
        n117 = Bundle By Name(cluster=w409, "Software Flags.Output Complete?"=TRUE) -> (w413:T8)
      }
      frame "-----------------INSTRUMENT HANDLE CLOSE----------------" {
      }
      frame "Abort session" {
        w424 = bool[] [] ("Software Flags.Advanced Seq Created?")
        # "Abort the session if it initiated"
        n118 = Unbundle By Name(w431) -> ("Software Flags"=w428:T10, "Channel Settings.Instrument handle"=w430:refnum<k15>[], "Channel Settings.Channel Number"=w429:string[])
        n119 = call "Abort Session.vi"("instrument handle"=w430, "Software Flags"=w428, "channel name"=w429, "error in (no error)"=w426) -> ("error out"=w427:errorcluster)  [unwired: 11 in]
        n120 = Bundle By Name(cluster=w431, "Software Flags.Advanced Seq Created?"=w424, "Software Flags.Initiated?"=w424, "Error Info.Error Phase"="Abort") -> (w425:T8)
        n121 = call <vilib>:"Clear Errors.vi"("error in (no error)"=w427) -> ("error out"=w422:errorcluster)  [unwired: 5 in, 1 out]
      }
      frame "Close Instrument Handle" {
        # "Close handle only if initialize is complete"
        # "Closing the instrument handle after power up/down"
        n122 = Unbundle By Name(w441) -> ("session reservation"=w432:refnum<class "Session Reservation.lvclass">, "Software Flags"=w434:T10, "Channel Settings.Instrument handle"=w440:refnum<k15>[])
        n123 = disable-structure shown="Enabled" {
          disable-tunnel: w440 -> [w445 _]
          disable-tunnel: [w444 w447] -> w439
          disable-tunnel: w437 -> [w443 w448]
          disable-tunnel: w434 -> [w442 _]
          disable-tunnel: w432 -> [_ w446]
          frame Disabled {
            n124 = call "Close Handle.vi"("instrument handle"=w445, "Software Flags"=w442, "error in (no error)"=w443) -> ("error out"=w444:errorcluster)  [unwired: 12 in]
          }
          frame Enabled {
            # "new session API will close sessions"
            n125 = call <vilib>:"Close Sessions.vi"("error in"=w448, "session reservation in"=w446) -> ("error out"=w450:errorcluster, "session reservation out"=w449:refnum<class "Session Reservation.lvclass">)  [unwired: 8 in]
            n126 = call <vilib>:"Unreserve Sessions.vi"("error in"=w450, "session reservation in"=w449) -> ("error out"=w447:errorcluster)  [unwired: 9 in]
          }
        }
        n127 = Merge Errors(w439, w437) -> (w438:errorcluster)
        n128 = Bundle By Name(cluster=w441, "Error Info.Error Phase"="Close Handle") -> (w436:T8)
      }
      frame "-------------- SAFE POWER DOWN--- -----------" {
      }
      frame "Safe Power Down" {
        # "Call the sequence which will safely power down all the pins"
        n129 = Unbundle By Name(w459) -> ("Measurement Configuration.Quick Power Down"=w455:bool, "Software Flags.PowerUp?"=w456:bool)
        n130 = case "Power Down?" shown="True" w456 {
          tunnel: [TRUE ("Power Down") w466] -> w457
          tunnel: w455 -> [_ w466]
          frame False {
            # "Power Down"
          }
          frame True {
            # "Power Up"
          }
        }
        n131 = case "Power Down?" shown="False" w457 {
          tunnel: w462 -> [w470 w477]
          tunnel: [w469 w475] -> w461
          tunnel: w460 -> [w467 w476]
          frame False {
            # "Sequence to powerdown the pins \nif there is an error during the power up/compliance limit is reached in between"
            n132 = for {
              tunnel: w467 -> [w474]
              shift-right: [w472] -> w469
              shift-left: w470 -> [w473]
              tunnel: string[] ["Abort session", "Reverse the Sequence", "Calculate total sequence time", "Configure Safe Power Down", "Configure Trigger", "Initiate", "Wait for complete", "Abort session", "Close Instrument Handle", "Update Error Message", "Exit"] -> [w471] mode=indexing
              n133 = Enqueue Element(queue=w474, element=w471, error in (no error)=w473) -> (error out=w472:errorcluster)  [unwired: 1 in, 2 out]
            }
          }
          frame True {
            # "Call emergency powerdown sequence"
            n134 = Enqueue Element(queue=w476, element="Emergency Power Down", error in (no error)=w477) -> (error out=w475:errorcluster)  [unwired: 1 in, 2 out]
          }
        }
        n135 = Bundle By Name(cluster=w459, "Error Info.Error Phase"="Safe Power Down", "Error Info.Error Code"=5001) -> (w464:T8)
      }
      frame "Reverse the Sequence" {
        # "In Case of power up, power should happen in the reverse sequence.\nHence reversing all the array which are needed for power down"
        n136 = call "Reverse Configurations for Safe PowerDown.vi"("Data Cluster"=w481, "error in (no error)"=w482) -> ("Data Cluster OUT"=w480:T8, "error out"=w483:errorcluster)  [unwired: 12 in]
      }
      frame "Configure Safe Power Down" {
        # "Configure the advanced sequence for power down using the controlled ramprate"
        n137 = Unbundle By Name(w498) -> ("Error Info.Error List"=w488:string[], "Measurement Configuration"=w494:T2, "Channel Settings.Instrument handle"=w497:refnum<k15>[], "Channel Settings.Channel Number"=w496:string[], "Ramp Configurations"=w495:T11)
        n138 = call "Configure Safe Power Down Sequence.vi"("Instrument handle IN"=w497, "Measurement Configuration"=w494, "Channel Name"=w496, "Ramp Configurations"=w495, "error in (no error)"=w491) -> ("Instrument Handle OUT"=w492:refnum<k15>[], "Advanced Sequence Created?"=w490:bool[], "error out"=w486:errorcluster)  [unwired: 8 in]
        n139 = Insert Into Array(array=w488, new element="Safe PowerDown Initiated" ("Error Message")) -> (w487:string[])  [unwired: 1 in]
        n140 = Bundle By Name(cluster=w498, "Error Info.Error List"=w487, "Error Info.Error Phase"="Safe Power Down", "Channel Settings.Instrument handle"=w492, "Software Flags.Advanced Seq Created?"=w490) -> (w493:T8)
      }
      frame "Wait for complete" {
        w510 = T17 1033 items=["Source Complete Event"=1030, "Measure Complete Event"=1031, "Sequence Iteration Complete Event"=1032, "Sequence Engine Done Event"=1033, "Pulse Complete Event"=1051, "Ready For Pulse Trigger Event"=1052] ("event")
        n141 = Unbundle By Name(w511) -> ("Ramp Configurations.Max Sequence Period Index"=w502:i32, "Channel Settings.Instrument handle"=w507:refnum<k15>[], "Channel Settings.Channel Number"=w505:string[], "Ramp Configurations.Total Sequence Time"=w506:dbl)
        n142 = Add(x=1.0, y=w506) -> (x+y=w501:dbl)
        n143 = Index Array(array=w507, index=w502) -> (element=w504:refnum<k15>)
        n144 = Index Array(array=w505, index=w502) -> (element=w503:string)
        n145 = call <instrlib>:"niDCPower Wait For Event With Channels.vi"("timeout (10.0)"=w501, "error in (no error)"=w508, "event"=w510, "channel name"=w503, "instrument handle"=w504) -> ("error out"=w509:errorcluster)  [unwired: 5 in, 1 out]
      }
      frame "---------------CANCEL IS PRESSED--------------" {
      }
      frame "Canceled" {
        # "Handle Cancel Event from Measurement UI (Safe Power down)"
        n146 = Unbundle By Name(w533) -> ("Software Flags.PowerUp?"=w518:bool, "Measurement Configuration.Quick Power Down"=w517:bool, "Error Info.Error List"=w523:string[], "Error Info.Error Phase"=w531:string)
        n147 = Flush Queue(queue=w529, error in (no error)=w527) -> (queue out=w530:refnum<queue>, error out=w528:errorcluster)  [unwired: 1 out]
        n148 = case "Power Down?" shown="False" w518 {
          tunnel: [TRUE ("Power Down") w535] -> w516
          tunnel: w517 -> [_ w535]
          frame False {
            # "Power Down"
          }
          frame True {
            # "Power Up"
          }
        }
        n149 = case shown="True" w516 {
          tunnel: w528 -> [w540 w554]
          tunnel: [w539 w553] -> w519
          tunnel: w530 -> [w537 w552]
          tunnel: w531 -> [w538 _]
          frame False {
            # "#dataLoggger"
            # "Call the appropriate sequence\nIf cancel is pressed"
            # "Power Up"
            n150 = case shown="\"Input Configuration\"" w538 {
              tunnel: [string[] ["Exit"] string[] ["Abort session", "Close Instrument Handle", "Exit"] string[] ["Emergency Power Down"] string[] ["Safe Power Down", "Stop Logger"] string[] ["Emergency Power Down"] string[] ["Abort session", "Close Instrument Handle", "Exit"]] -> w536
              frame "Close Handle", "Init", "Input Validation" {
              }
              frame "Input Configuration" {
              }
              frame "Abort" {
              }
              frame "Measure", "Power UP", "Verify Sequence" {
              }
              frame "Safe Power Down" {
              }
              frame Default {
              }
            }
            n151 = for {
              shift-right: [w543] -> w539
              shift-left: w540 -> [w544]
              tunnel: w537 -> [w542]
              tunnel: w536 -> [w541] mode=indexing
              n152 = Enqueue Element(queue=w542, element=w541, error in (no error)=w544) -> (error out=w543:errorcluster)  [unwired: 1 in, 2 out]
            }
          }
          frame True {
            # "Power Down - Call the reset state"
            n153 = for {
              tunnel: w552 -> [w556]
              shift-right: [w557] -> w553
              shift-left: w554 -> [w558]
              tunnel: string[] ["Emergency Power Down", "Stop Logger"] -> [w555] mode=indexing
              n154 = Enqueue Element(queue=w556, element=w555, error in (no error)=w558) -> (error out=w557:errorcluster)  [unwired: 1 in, 2 out]
            }
          }
        }
        n155 = call "Error Message.vi"("Error Code"=5000 ("Error Info.Error Code"), "error in (no error)"=w519) -> ("Error Message"=w524:string, "error out"=w520:errorcluster)  [unwired: 11 in, 1 out]
        n156 = Insert Into Array(array=w523, index=0, new element=w524) -> (w522:string[])
        n157 = Bundle By Name(cluster=w533, "Software Flags.Canceled?"=TRUE, "Error Info.Error List"=w522) -> (w532:T8)
      }
      frame "-------------- EMERGENCY POWER DOWN--------------" {
      }
      frame "Emergency Power Down" {
        # "Emeregency Power Down will be called if there is an error during Safe Power Down / Error in Power Down"
        n158 = Unbundle By Name(w568) -> ("Measurement Configuration.Quick Power Down"=w564:bool, "Software Flags.PowerUp?"=w565:bool)
        n159 = for {
          tunnel: w574 -> [w580]
          shift-right: [w578] -> w572
          shift-left: w571 -> [w579]
          tunnel: string[] ["Abort session", "Reset the Instrument", "Close Instrument Handle", "Update Error Message", "Exit"] -> [w577] mode=indexing
          n160 = Enqueue Element(queue=w580, element=w577, error in (no error)=w579) -> (error out=w578:errorcluster)  [unwired: 1 in, 2 out]
        }
        n161 = case "Power Down?" shown="True" w565 {
          tunnel: [TRUE ("Power Down") w576] -> w563
          tunnel: w564 -> [_ w576]
          frame False {
            # "Power Down"
          }
          frame True {
            # "Power Up"
          }
        }
        n162 = Select(t=5018 ("Error Info.Error Code"), s=w563, f=5002 ("Error Info.Error Code")) -> (s? t:f=w569:i32)
        n163 = Bundle By Name(cluster=w568, "Error Info.Error Code"=w569) -> (w570:T8)
      }
      frame "Reset the Instrument" {
        # "Reset the is Safe Power down is failed"
        n164 = Unbundle By Name(w601) -> ("Measurement Configuration.Quick Power Down"=w585:bool, "Software Flags.PowerUp?"=w586:bool, "Error Info.Error Occurred?"=w590:bool, "Error Info.Error Code"=w596:i32, "Channel Settings.Instrument handle"=w600:refnum<k15>[], "Channel Settings.Channel Number"=w599:string[])
        n165 = for {
          tunnel: w600 -> [w607] mode=indexing
          tunnel: w599 -> [w606] mode=indexing
          tunnel: w591 -> [w605]
          tunnel: [w604] -> w598 mode=indexing
          n166 = call <instrlib>:"niDCPower Reset With Channels.vi"("error in (no error)"=w605, "channel name"=w606, "instrument handle"=w607) -> ("error out"=w604:errorcluster)  [unwired: 7 in, 1 out]
        }
        n167 = case "Power Down?" shown="True" w586 {
          tunnel: [TRUE ("Power Down") w603] -> w584
          tunnel: w585 -> [_ w603]
          frame False {
            # "Power Down"
          }
          frame True {
            # "Power Up"
          }
        }
        n168 = Merge Errors(w598) -> (w597:errorcluster)
        n169 = Unbundle(w597) -> ("status"=w589:bool)  [unwired: 2 out]
        n170 = Select(t=5019 ("f"), s=w584, f=5003 ("t")) -> (s? t:f=w587:i32)
        n171 = Or(x=w590, y=w589) -> (x .or. y?=w588:bool)
        n172 = call <vilib>:"Clear Errors.vi"("error in (no error)"=w597) -> ("error out"=w593:errorcluster)  [unwired: 5 in, 1 out]
        n173 = Select(t=w587, s=w589, f=w596) -> (s? t:f=w594:i32)
        n174 = Bundle By Name(cluster=w601, "Error Info.Error Code"=w594, "Error Info.Error Occurred?"=w588) -> (w595:T8)
        n175 = Merge Errors(w593, w591) -> (w592:errorcluster)
      }
      frame "----------- MISCELLANEOUS -------------" {
      }
      frame "Error" {
        # "Capture errors and route to error handling"
        n176 = Unbundle By Name(w624) -> ("Error Info.Error Phase"=w623:string, "Log.Log Data?"=w613:bool)
        n177 = Unbundle(w616) -> ("code"=w614:i32, "source"=w615:string)  [unwired: 1 out]
        n178 = call <vilib>:"Clear Errors.vi"("error in (no error)"=w616) -> ("error out"=w619:errorcluster)  [unwired: 5 in, 1 out]
        n179 = case shown="5000..5200" w614 {
          tunnel: w624 -> [w630 w633]
          tunnel: [w629 w632] -> w617
          tunnel: w615 -> [w628 _]
          frame Default {
            # "LabVIEW Error"
            n180 = Unbundle By Name(w630) -> ("Error Info.Error List"=w626:string[])
            n181 = Insert Into Array(array=w626, new element=w628) -> (w625:string[])  [unwired: 1 in]
            n182 = Bundle By Name(cluster=w630, "Error Info.Error Occurred?"=TRUE, "Error Info.Error List"=w625) -> (w629:T8)
          }
          frame 5000..5200 {
            # "Custom error"
            n183 = Bundle By Name(cluster=w633, "Error Info.Error Occurred?"=TRUE) -> (w632:T8)
          }
        }
        n184 = Flush Queue(queue=w621, error in (no error)=w619) -> (queue out=w620:refnum<queue>, error out=w618:errorcluster)  [unwired: 1 out]
        n185 = case shown="\"Close Handle\"" w623 {
          tunnel: w618 -> [w637 w645 w649 w660 w668 w676 w682 w691 w699]
          tunnel: w620 -> [w636 w644 w648 w658 w666 w674 w683 w689 w698]
          tunnel: [w635 w643 w647 w659 w667 w675 w681 w690 w697] -> w622
          tunnel: w613 -> [_ _ _ w654 _ _ w678 _ _]
          tunnel: w612 -> [_ _ _ _ _ _ _ _ _]
          frame Default {
            n186 = for {
              tunnel: w636 -> [w640]
              shift-right: [w639] -> w635
              shift-left: w637 -> [w641]
              tunnel: string[] ["Abort session", "Close Instrument Handle", "Exit"] -> [w638] mode=indexing
              n187 = Enqueue Element(queue=w640, element=w638, error in (no error)=w641) -> (error out=w639:errorcluster)  [unwired: 1 in, 2 out]
            }
          }
          frame "Init", "Input Validation" {
            n188 = Enqueue Element(queue=w644, element="Exit", error in (no error)=w645) -> (error out=w643:errorcluster)  [unwired: 1 in, 2 out]
          }
          frame "Input Configuration" {
            n189 = for {
              tunnel: w648 -> [w652]
              shift-right: [w651] -> w647
              shift-left: w649 -> [w653]
              tunnel: string[] ["Abort session", "Close Instrument Handle", "Exit"] -> [w650] mode=indexing
              n190 = Enqueue Element(queue=w652, element=w650, error in (no error)=w653) -> (error out=w651:errorcluster)  [unwired: 1 in, 2 out]
            }
          }
          frame "Power UP" {
            n191 = Select(t=string[] ["Safe Power Down", "Stop Logger"], s=w654, f=string[] ["Safe Power Down"]) -> (s? t:f=w656:string[])
            n192 = for {
              shift-right: [w663] -> w659
              shift-left: w660 -> [w664]
              tunnel: w656 -> [w662] mode=indexing
              tunnel: w658 -> [w661]
              n193 = Enqueue Element(queue=w661, element=w662, error in (no error)=w664) -> (error out=w663:errorcluster)  [unwired: 1 in, 2 out]
            }
          }
          frame "Verify Sequence" {
            n194 = for {
              shift-right: [w671] -> w667
              shift-left: w668 -> [w672]
              tunnel: string[] ["Safe Power Down"] -> [w670] mode=indexing
              tunnel: w666 -> [w669]
              n195 = Enqueue Element(queue=w669, element=w670, error in (no error)=w672) -> (error out=w671:errorcluster)  [unwired: 1 in, 2 out]
            }
          }
          frame "Safe Power Down" {
            # "Enqueue Safe Power Down States"
            n196 = Enqueue Element(queue=w674, element="Emergency Power Down", error in (no error)=w676) -> (error out=w675:errorcluster)  [unwired: 1 in, 2 out]
          }
          frame "Measure" {
            n197 = Select(t=string[] ["Safe Power Down", "Stop Logger"], s=w678, f=string[] ["Safe Power Down"]) -> (s? t:f=w680:string[])
            n198 = for {
              shift-right: [w686] -> w681
              shift-left: w682 -> [w687]
              tunnel: w680 -> [w685] mode=indexing
              tunnel: w683 -> [w684]
              n199 = Enqueue Element(queue=w684, element=w685, error in (no error)=w687) -> (error out=w686:errorcluster)  [unwired: 1 in, 2 out]
            }
          }
          frame "Abort" {
            n200 = for {
              tunnel: w689 -> [w693]
              shift-right: [w694] -> w690
              shift-left: w691 -> [w695]
              tunnel: string[] ["Abort session", "Close Instrument Handle", "Exit"] -> [w692] mode=indexing
              n201 = Enqueue Element(queue=w693, element=w692, error in (no error)=w695) -> (error out=w694:errorcluster)  [unwired: 1 in, 2 out]
            }
          }
          frame "Close Handle" {
            n202 = Enqueue Element At Opposite End(queue=w698, element="Exit", error in (no error)=w699) -> (error out=w697:errorcluster)  [unwired: 1 in, 2 out]
          }
        }
      }
      frame "Update Error Message" {
        n203 = Unbundle By Name(w708) -> ("Error Info.Error List"=w702:string[], "Error Info.Error Code"=w707:i32)
        n204 = call "Error Message.vi"("Error Code"=w707, "error in (no error)"=w706) -> ("Error Message"=w703:string, "error out"=w705:errorcluster)  [unwired: 11 in, 1 out]
        n205 = Insert Into Array(array=w702, new element=w703) -> (w701:string[])  [unwired: 1 in]
        n206 = Bundle By Name(cluster=w708, "Error Info.Error List"=w701) -> (w704:T8)
      }
      frame "Exit" {
        w738 = TRUE  # Stop Core Logic Loop
        # "Exit Core Logic and raise errors if any"
        n207 = Unbundle By Name(w719) -> ("Software Flags.Canceled?"=w726:bool, "Error Info.Error Occurred?"=w727:bool, "Error Info.Error List"=w724:string[], "session reservation"=w711:refnum<class "Session Reservation.lvclass">)
        n208 = Flush Queue(queue=w733) -> (queue out=w734:refnum<queue>, error out=w737:errorcluster)  [unwired: 1 in, 1 out]
        n209 = Send Notification(notification=TRUE, notifier=w736) -> (error out=w729:errorcluster)  [unwired: 1 in, 1 out]
        n210 = Release Queue(queue=w734, error in (no error)=w737) -> (error out=w731:errorcluster)  [unwired: 1 in, 2 out]
        n211 = Merge Errors(w729, w731, w730) -> (w732:errorcluster)
        n212 = Not(x=w727) -> (.not. x?=w728:bool)
        n213 = And(x=w726, y=w728) -> (x .and. y?=w725:bool)
        n214 = case "Cancelled?" shown="False" w725 {
          tunnel: w732 -> [w746 w755]
          tunnel: [w745 w754] -> w716
          tunnel: w727 -> [w744 _]
          tunnel: w724 -> [w743 _]
          frame False {
            n215 = case shown="True" w744 {
              tunnel: w746 -> [w747 w752]
              tunnel: [w747 w751] -> w745
              tunnel: w743 -> [_ w748]
              frame False {
                # "No Error to raise"
              }
              frame True {
                # "Raise error to measurement link"
                n216 = call "Form Error Message.vi"("Error Message"=w748, "error code (0)"=5090, "Error?"=TRUE, "error in (no error)"=w752) -> ("error out"=w751:errorcluster)  [unwired: 11 in]
              }
            }
          }
          frame True {
            # "Notify user that\ncancel is pressed"
            n217 = call "Generate Error.vi"("Error Code"=5000, "error in (no error)"=w755) -> ("error out"=w754:errorcluster)  [unwired: 13 in]
          }
        }
        n218 = call <vilib>:"Clear Errors.vi"("error in (no error)"=w716) -> ("error out"=w712:errorcluster)  [unwired: 5 in, 1 out]
        n219 = call <vilib>:"Close Sessions.vi"("error in"=w712, "session reservation in"=w711) -> ("error out"=w714:errorcluster, "session reservation out"=w713:refnum<class "Session Reservation.lvclass">)  [unwired: 8 in]
        n220 = Unbundle By Name(w719) -> ("Log.User Event"=w723:refnum<user-event>, "Log.Log Data?"=w722:bool, "Measurement Configuration.Data Capture"=w721:bool)
        n221 = call <vilib>:"Unreserve Sessions.vi"("error in"=w714, "session reservation in"=w713) -> ("error out"=w710:errorcluster)  [unwired: 9 in]
        n222 = call <vilib>:"Clear Errors.vi"("error in (no error)"=w710) -> ("error out"=w709:errorcluster)  [unwired: 5 in, 1 out]
        n223 = And(x=w722, y=w721) -> (x .and. y?=w720:bool)
        n224 = case shown="False" w720 {
          tunnel: w709 -> [w739 w742]
          tunnel: [w739 w741] -> w718
          tunnel: w723 -> [_ w740]
          frame False {
          }
          frame True {
            n225 = Destroy User Event(user event=w740, error in=w742) -> (error out=w741:errorcluster)
          }
        }
        n226 = Merge Errors(w716, w718) -> (w717:errorcluster)
      }
    }
  }
  n227 = while {
    shift-right: [w761] -> w18
    shift-left: w13 -> [w766]
    shift-right: [w764] -> _
    shift-left: "Init" -> [w765]
    tunnel: "Measurement Context In" -> [w763]
    tunnel: w12 -> [w759]
    shift-right: [w757] -> _
    shift-left: w10 -> [w758]
    tunnel: w8 -> [w756]
    stop <- w760 stop-if-true
    # "Events Loop (Controls core logic flow and Monitors events from Measurement Link)"
    n228 = case shown="\"\"" w765 {
      selector: w765 -> [w770 _ _ _ _ _ _ _]
      tunnel: w766 -> [w773 w779 w786 w792 w796 w806 w808 w815]
      tunnel: [w771 w779 w785 w791 w796 w805 w808 w813] -> w761
      tunnel: ["" "" w787 "" _ w801 _ _] -> w764
      tunnel: w763 -> [_ _ _ _ _ w804 _ _]
      tunnel: [_ _ _ TRUE _ _ _ _] -> w762
      tunnel: w759 -> [_ _ w784 w789 _ _ _ _]
      tunnel: w758 -> [w775 w777 w781 w790 w795 w798 w807 _]
      tunnel: [w775 w777 w781 w790 w795 w798 w807 TRUE ("Enable Checks?")] -> w757
      tunnel: w756 -> [_ _ _ _ _ _ _ w810]
      frame Default {
        w767 = 5004 ("error code (0)")
        # "Unknow case handling"
        n229 = call "Error Message.vi"("Error Code"=w767) -> ("Error Message"=w768:string)  [unwired: 12 in, 2 out]
        n230 = Format Into String(format string=w768, error in=w773, w770, "Event Loop" ("input 2")) -> (resulting string=w774:string, error out=w772:errorcluster)  [unwired: 1 in]
        n231 = call <vilib>:"Error Cluster From Error Code.vi"("error in (no error)"=w772, "error message (\"\")"=w774, "error code (0)"=w767) -> ("error out"=w771:errorcluster)  [unwired: 6 in]
      }
      frame "Init" {
        # "Place Holder for any initializes in events loop"
      }
      frame "" {
        # "Checks if core logic flow ended"
        # "Checks whether the core logic is finished"
        n232 = Wait on Notification(notifier=w784, timeout in ms (-1)=50, error in (no error)=w786) -> (notification=w782:bool, error out=w785:errorcluster)  [unwired: 1 in, 2 out]
        n233 = Select(t="Exit", s=w782, f="Check Cancel") -> (s? t:f=w787:string)
      }
      frame "Exit" {
        # "Exit Events monitoring loop"
        n234 = Release Notifier(notifier=w789, error in (no error)=w792) -> (error out=w791:errorcluster)  [unwired: 1 in, 2 out]
      }
      frame "-------- Events Monitoring --------" {
      }
      frame "Check Cancel" {
        # "To avoid canceled cases to be added more than once"
        # "Redirect to following event monitoring (if any)"
        # "Checks if the user click Stop button in instrument studio"
        n235 = property class="Measure Call Context.lvclass"(reference=w804, error in=w806) -> (error out=w805:errorcluster, "Accessor:Is Canceled"=w799:bool)  [unwired: 1 out]
        n236 = Not(x=w798) -> (.not. x?=w797:bool)
        n237 = And(x=w797, y=w799) -> (x .and. y?=w800:bool)
        n238 = Select(t="Canceled", s=w800, f="") -> (s? t:f=w801:string)
      }
      frame "---------- Event Actions -----------" {
      }
      frame "Canceled" {
        # "Redirect Core Logic Flow to Safe Power Down"
        n239 = Flush Queue(queue=w810, error in (no error)=w815) -> (queue out=w809:refnum<queue>, error out=w814:errorcluster)  [unwired: 1 out]
        n240 = Enqueue Element(queue=w809, element="Canceled" ("State In"), error in (no error)=w814) -> (error out=w813:errorcluster)  [unwired: 1 in, 2 out]
      }
    }
    n241 = Or(x=w761, y=w762) -> (x .or. y?=w760:bool)
  }
  n242 = Merge Errors(w4, w18) -> (→"error out":errorcluster)
  "Measurement Context Out" <- "Measurement Context In"
